vi "Reanimate -Simple.vi"() -> ()   [LabVIEW 2017]
doc: "A demonstration of reanimating the Corpse (legacy) at the grave (Diagram Disable Structure). This includes step-by-step instructions for enabling the Corpse (legacy) frame and disabling the Spirit (refactored) frame for the grave with one of two methods: shortcut menu plugin or Quick Drop shortcut plugin."
panel:
  out "Any?":bool
  in  "Input":bool[](array[boolean])=[FALSE, FALSE, FALSE, FALSE, FALSE, FALSE, TRUE, FALSE, FALSE, FALSE]
  # "Overview: Demonstrates reanimating (enabling) the legacy code\nInstructions:\n1. Run the VI\n2. Observe the value of the Any? indicator\n3. Uncheck the TRUE element in the Input array\n4. Run the VI\n5. Observe the value of the Any? indicator\n6. Switch to the block diagram and follow the instructions to use the legacy code instead of refactored code"
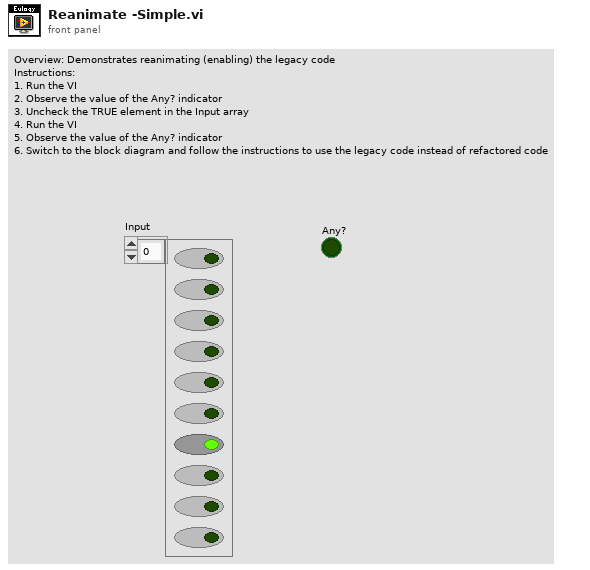
[diagram p1: front panel]
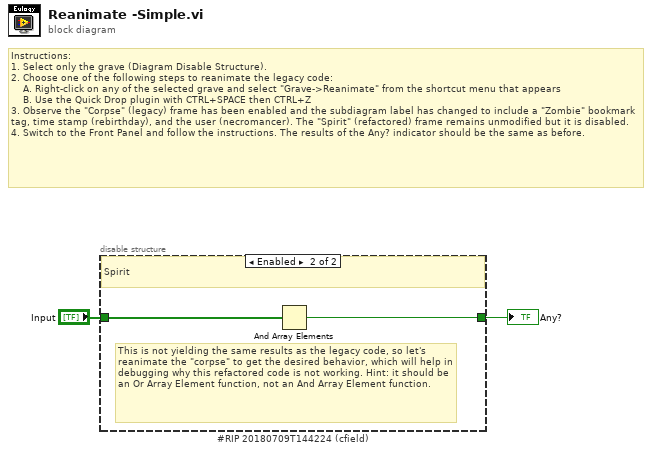
[diagram p0: block diagram]
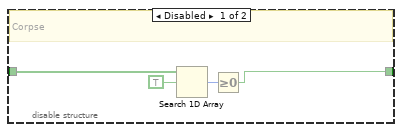
[diagram p2: hidden frame]
diagram:
  # "Instructions:\n1. Select only the grave (Diagram Disable Structure).\n2. Choose one of the following steps to reanimate the legacy code:\n    A. Right-click on any of the selected grave and select \"Grave->Reanimate\" from the shortcut menu that appears\n    B. Use the Quick Drop plugin with CTRL+SPACE then CTRL+Z\n3. Observe the \"Corpse\" (legacy) frame has been enabled and the subdiagram label has changed to include a \"Zombie\" bookmark tag, time stamp (rebirthday), and the user (necromancer). The \"Spirit\" (refactored) frame remains unmodified but it is disabled.\n4. Switch to the Front Panel and follow the instructions. The results of the Any? indicator should be the same as before."
  n1 = disable-structure "#RIP 20180709T144224 (cfield)" shown="Enabled" {
    disable-tunnel: "Input" -> [w6 w8]
    disable-tunnel: [w5 w7] -> w1
    frame Disabled {
      # "Corpse"
      n2 = Search 1D Array(1D array=w6, element=TRUE) -> (index of element=w3:i32)  [unwired: 1 in]
      n3 = Greater Or Equal To 0?(x=w3) -> (x >= 0?=w5:bool)
    }
    frame Enabled {
      # "This is not yielding the same results as the legacy code, so let's reanimate the \"corpse\" to get the desired behavior, which will help in debugging why this refactored code is not working. Hint: it should be an Or Array Element function, not an And Array Element function."
      # "Spirit"
      n4 = And Array Elements(Boolean array=w8) -> (logical AND=w7:bool)
    }
  }
  "Any?" <- w1
